vi "kill_agent.vi"(0 "Host_Reference":refnum<class "HGF_Reference.lvclass">, 2 "timeout in ms (-1)":i32=-1, 5 "error in (no error)":errorcluster) -> (14 "dup Host_Reference":refnum<class "HGF_Reference.lvclass">, 16 "dup timeout in ms (-1)":i32=-1, 19 "error out":errorcluster)   [LabVIEW 2009, in "MoAgSy.lvlib" / "MoAgSy_Host.lvclass"]
doc: "<B>public</B> GUI for killing Agents.\n<B>Frontpanel has to be shown at VI call.</B>\n\nF.Berck@gsil.de\nGSI Darmstadt 2009"
uses:
  MoAgSy_Host.lvclass
  HGF_BaseClasses/HGF_Reference/HGF_Reference.lvclass
panel:
  in  "abort":bool
  in  "killAgent":bool
  in  "AgentSelect":u16(ring)
  # "Select Agent to kill"
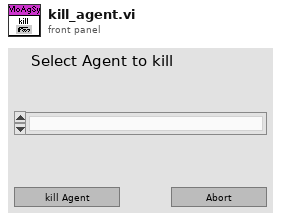
[diagram p1: front panel]
types:
  T1 = cluster{"killNotifier":refnum<notifier>, "Agent ID":string}[]
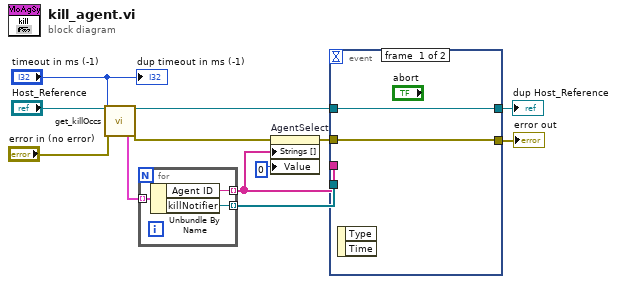
[diagram p0: block diagram]
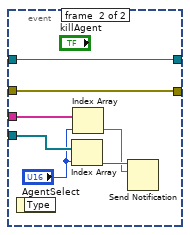
[diagram p2: hidden frame]
diagram:
  n1 = call "get_killOccs.vi"("Host_Reference"="Host_Reference", "timeout in ms (-1)"="timeout in ms (-1)", "error in (no error)"="error in (no error)") -> ("dup Host_Reference"=w10:refnum<class "HGF_Reference.lvclass">, "Kill Occs"=w7:T1, "error out"=w6:errorcluster)  [unwired: 14 out]
  n2 = for {
    tunnel: w7 -> [w15] mode=indexing
    tunnel: [w14] -> w2 mode=indexing
    tunnel: [w13] -> w4 mode=indexing
    n3 = Unbundle By Name(w15) -> ("Agent ID"=w14:string, "killNotifier"=w13:refnum<notifier>)
  }
  n4 = property on="AgentSelect" class="Ring (strict)"(error in=w6, "Strings []"=w2, "Value"=0) -> (error out=w5:errorcluster)  [unwired: 1 in, 1 out]
  n5 = event shown="[1] \"killAgent\": Value Change" {
    selector: _ -> [_ _]
    dyn-events: _ -> [_ _]
    timeout: _ -> [_ _]
    tunnel: w10 -> [w17 w23]
    tunnel: [w17 w23] -> w9
    tunnel: w5 -> [w16 w22]
    tunnel: [w16 w22] -> w8
    tunnel: w4 -> [_ w24]
    tunnel: w2 -> [_ w21]
    event #0 {
      n6 = event-data() -> ()  [unwired: 3 out]
    }
    event #1 {
      n7 = event-data() -> ()  [unwired: 2 out]
      n8 = Index Array(array=w24, index="AgentSelect") -> (element=w19:refnum<notifier>)
      n9 = Index Array(array=w21, index="AgentSelect") -> (element=w18:string)
      n10 = Send Notification(notification=w18, notifier=w19) -> ()  [unwired: 1 in, 2 out]
    }
  }
  "dup Host_Reference" <- w9
  "error out" <- w8
  "dup timeout in ms (-1)" <- "timeout in ms (-1)"
